vi "Exp_SetExposuresPerFrame.vi"(8 "error in (no error)":errorcluster, 10 "Exposures Per Frame":i32, 11 "LightField Automation in":refnum<class "LightField Automation.lvclass">) -> (0 "error out":errorcluster, 3 "LightField Automation out":refnum<class "LightField Automation.lvclass">)   [LabVIEW 2019, in "LightField Automation.lvclass"]
uses:
  LightField Automation.lvclass
  C:/Program Files/Princeton Instruments/LightField/PrincetonInstruments.LightFieldAddInSupportServices.dll
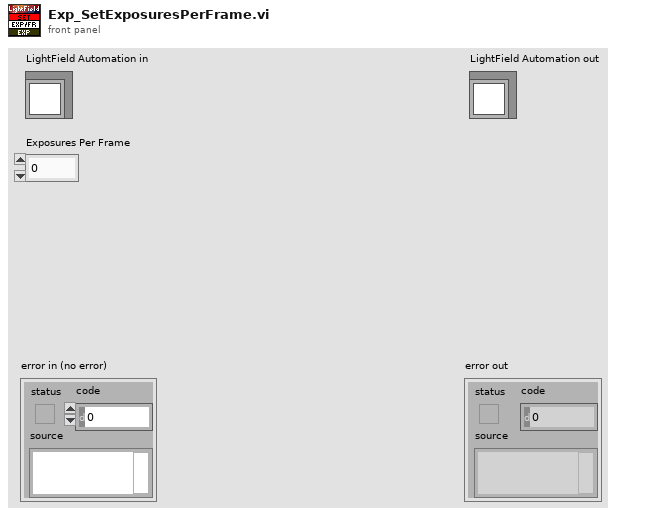
[diagram p1: front panel]
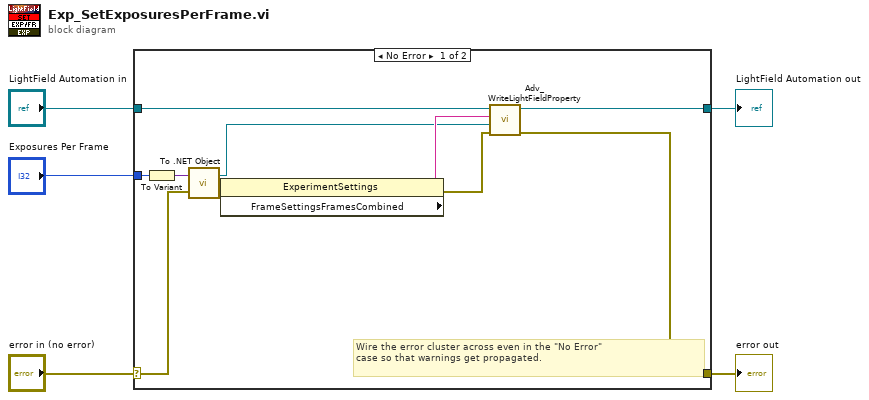
[diagram p0: block diagram]
diagram:
  n1 = case shown="No Error" "error in (no error)" {
    selector: "error in (no error)" -> [w13 w17]
    tunnel: [w6 w17] -> w4
    tunnel: [w10 w16] -> w2
    tunnel: "LightField Automation in" -> [w11 w16]
    tunnel: "Exposures Per Frame" -> [w14 _]
    frame No Error {
      # "Wire the error cluster across even in the \"No Error\"\ncase so that warnings get propagated."
      n2 = To Variant(anything=w14) -> (Variant=w15:variant)
      n3 = call <vilib>:"To .NET Object.vi"("error in (no error)"=w13, "anything"=w15) -> ("error out"=w12:errorcluster, ".NET object"=w7:refnum<k24>)
      n4 = property class="ExperimentSettings"(error in=w12) -> (error out=w9:errorcluster, "FrameSettingsFramesCombined"=w8:string)  [unwired: 1 in, 1 out]
      n5 = call "Adv_WriteLightFieldProperty.vi"("error in (no error)"=w9, "value"=w7, "setting"=w8, "LightField Automation in"=w11) -> ("error out"=w6:errorcluster, "LightField Automation out"=w10:refnum<class "LightField Automation.lvclass">)  [unwired: 6 in]
    }
    frame Error {
    }
  }
  "error out" <- w4
  "LightField Automation out" <- w2
